vi "PH_Powermeter_BaseClass.PC Set Trigger Level.vi"(0 "VI in":refnum<vi>, 2 "Wanted Trigger Level [%]":dbl=2.0, 5 "error in (no error)":errorcluster) -> (14 "VI out":refnum<vi>, 19 "error out":errorcluster)   [LabVIEW 2014, in "PH_Powermeter_BaseClass.lvlib"]
doc: "If the incoming value is not zero and deiffers from stored value, the scaling factor is set to own attributtes. Aferwards, the energy is recalculated and set as well to own attributes as to GUI and DIM service."
uses:
  PH_Powermeter_BaseClass.lvlib
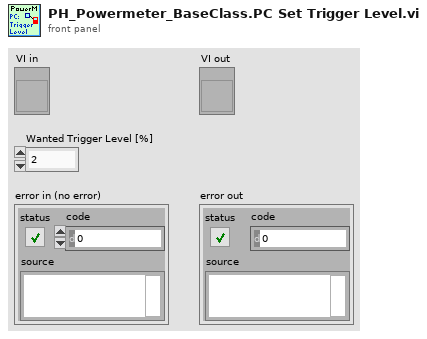
[diagram p1: front panel]
types:
  T1 = typedef "PH_Powermeter_BaseClass.lvlib/PH_Powermeter_BaseClass.i attribute.ctl" = cluster{"GUI References":T2, "Connection":T3, "Head Attributes":T5, "VISA resource":refnum<visa-resource-name>, "Energy":T6, "Service ID Energy":i32, "Wanted Settings":T7, "Current Settings":T7}
  T2 = typedef "PH_Powermeter_BaseClass.lvlib/PH_Powermeter_BaseClass.GUI Refs.ctl" = cluster{"Head Attributes":refnum<vi>, "Energy":refnum<vi>, "Connection":refnum<vi>, "VISA Resource":refnum<vi>, "Scaling Factor":refnum<vi>, "Range":refnum<vi>, "Wavelength":refnum<vi>, "Trigger Level":refnum<vi>, "Wanted Settings":refnum<vi>, "Current Settings":refnum<vi>}
  T3 = typedef "PH_Powermeter_BaseClass.lvlib/PH_Powermeter_BaseClass.Connection.ctl" = cluster{"failed checks":i8, "Timeout":bool, "Data read":string, "Failure":bool, "Error":bool, "State":T4}
  T4 = typedef "PH_Powermeter_BaseClass.lvlib/PH_Powermeter_BaseClass.State.ctl" = enum32{"off", "operating", "opened", "checked", "connected", "Sets to change", "running"}
  T5 = typedef "PH_Powermeter_BaseClass.lvlib/PH_Powermeter_BaseClass.Head Attributes.ctl" = cluster{"Instrument Type":string, "Head Version":string, "Head Name":string, "Serial Number":string, "Firmware":string, "Sensor Type":string, "MinimumRange":u32, "Maximum Range":u32, "Min Wavelength":i32, "Max Wavelength":i32}
  T6 = typedef "PH_Powermeter_BaseClass.lvlib/PH_Powermeter_BaseClass.Energy.ctl" = cluster{"current Value":dbl, "unscaled":dbl, "Scaling Factor":dbl}
  T7 = typedef "PH_Powermeter_BaseClass.lvlib/PH_gentec_BaseClass.Head Settings.ctl" = cluster{"Trigger Level":dbl, "Wavelength":u32, "Range":u32}
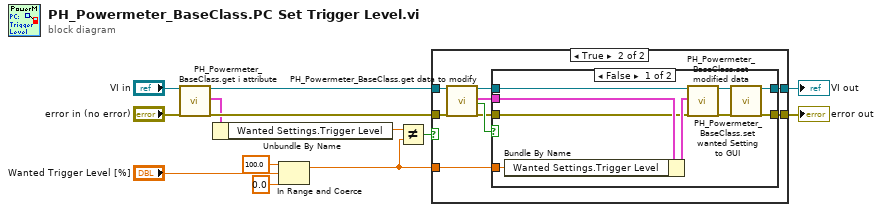
[diagram p0: block diagram]
diagram:
  n1 = call "PH_Powermeter_BaseClass.get i attribute.vi"("i ref in"="VI in", "error in (no error)"="error in (no error)") -> ("i ref out"=w8:refnum<vi>, "i attribute"=w7:T1, "error out"=w9:errorcluster)  [unwired: 15 in]
  n2 = Unbundle By Name(w7) -> ("Wanted Settings.Trigger Level"=w6:dbl)
  n3 = In Range and Coerce(upper limit=100.0, x="Wanted Trigger Level [%]", lower limit=0.0) -> (coerced(x)=w3:dbl)  [unwired: 1 out]
  n4 = Not Equal?(x=w6, y=w3) -> (x != y?=w5:bool)
  n5 = case shown="True" w5 {
    tunnel: [w14 w22] -> w13
    tunnel: [w15 w20] -> w11
    tunnel: w9 -> [w14 w18]
    tunnel: w8 -> [w15 w17]
    tunnel: w3 -> [_ w16]
    frame False {
    }
    frame True {
      n6 = call "PH_Powermeter_BaseClass.get data to modify.vi"("i ref in"=w17, "error in (no error)"=w18) -> ("i ref out"=w19:refnum<vi>, "i attribute"=w24:T1, "timed out"=w23:bool, "error out"=w21:errorcluster)  [unwired: 14 in]
      n7 = case shown="False" w23 {
        tunnel: w19 -> [w33 w35]
        tunnel: [w27 w35] -> w20
        tunnel: w21 -> [w29 w34]
        tunnel: [w25 w34] -> w22
        tunnel: w24 -> [w31 _]
        tunnel: w16 -> [w30 _]
        frame False {
          n8 = Bundle By Name(cluster=w31, "Wanted Settings.Trigger Level"=w30) -> (w32:T1)
          n9 = call "PH_Powermeter_BaseClass.set modified data.vi"("i ref in"=w33, "i attribute"=w32, "error in (no error)"=w29) -> ("i ref out"=w28:refnum<vi>, "error out"=w26:errorcluster)  [unwired: 15 in]
          n10 = call "PH_Powermeter_BaseClass.set wanted Setting to GUI.vi"("VI in"=w28, "error in (no error)"=w26) -> ("VI out"=w27:refnum<vi>, "error out"=w25:errorcluster)  [unwired: 16 in]
        }
        frame True {
        }
      }
    }
  }
  "error out" <- w13
  "VI out" <- w11
